vi "Main_PC.vi"() -> ()   [LabVIEW 2019]
uses:
  <vilib>/myRIO/Instrument Drivers/Onboard IO/UART/typedef/VISA Configuration.ctl
  <vilib>/Instr/_visa.llb/VISA Configure Serial Port (Instr).vi
  <vilib>/myRIO/Instrument Drivers/Onboard IO/UART/UART.lvlib
panel:
  in  "VISA resource name":refnum<visa-resource-name>
  out "Drilling Process":string
  out "RollDetection":bool
  out "Ready to Fly":bool
  in  "stop":bool
  out "error out":errorcluster
  in  "error in (no error)":errorcluster
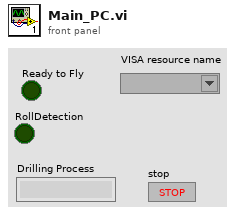
[diagram p1: front panel]
types:
  T1 = typedef "UART.lvlib/VISA Configuration.ctl" = cluster{"baud rate (9600)":u32, "data bits (8)":u16, "parity (0:none)":enum16{"None", "Odd", "Even", "Mark", "Space"}, "stop bits (10: 1 bit)":u16, "flow control (0:none)":u16, "termination char\n(0xA = '\\n' = LF) ":u8, "Enable Termination\nChar (T)":bool, "timeout (10sec)":u32}
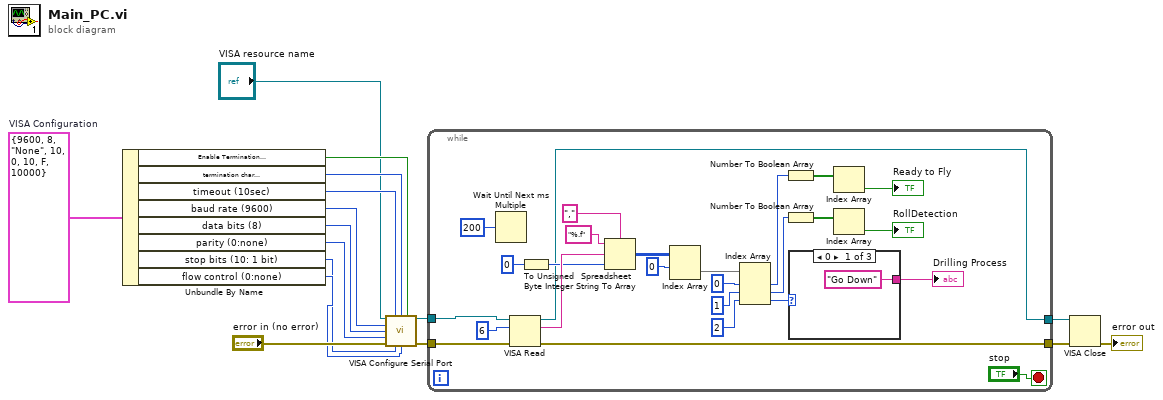
[diagram p0: block diagram]
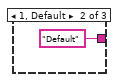
[diagram p2: hidden frame]
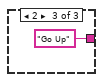
[diagram p3: hidden frame]
diagram:
  w4 = T1 {"baud rate (9600)"=9600, "data bits (8)"=8, "parity (0:none)"=enum."None", "stop bits (10: 1 bit)"=10, "flow control (0:none)"=0, "termination char\n(0xA = '\\n' = LF) "=10, "Enable Termination\nChar (T)"=FALSE, "timeout (10sec)"=10000}  # VISA Configuration
  n1 = Unbundle By Name(w4) -> ("Enable Termination\nChar (T)"=w13:bool, "termination char\n(0xA = '\\n' = LF)"=w12:u8, "timeout (10sec)"=w11:u32, "baud rate (9600)"=w6:u32, "data bits (8)"=w7:u16, "parity (0:none)"=w8:enum16{"None", "Odd", "Even", "Mark", "Space"}, "stop bits (10: 1 bit)"=w9:u16, "flow control (0:none)"=w10:u16)
  n2 = call-poly "VISA Configure Serial Port"("VISA resource name"="VISA resource name", "timeout (10sec)"=w11, "termination char\n(0xA = '\\n' = LF)"=w12, "Enable Termination\nChar (T)"=w13, "baud rate (9600)"=w6, "data bits (8)"=w7, "parity (0:none)"=w8, "error in (no error)"="error in (no error)", "stop bits (10: 1 bit)"=w9, "flow control (0:none)"=w10) -> ("VISA resource name out"=w15:refnum<visa-resource-name>, "error out"=w14:errorcluster)  [unwired: 4 in]
  n3 = while {
    tunnel: w15 -> [w19]
    tunnel: w14 -> [w41]
    tunnel: [w40] -> w2
    tunnel: [w17] -> w3
    stop <- "stop" stop-if-true
    n4 = Wait Until Next ms Multiple(millisecond multiple=u32 200) -> ()  [unwired: 1 out]
    n5 = VISA Read(VISA resource name=w19, byte count=u32 6 ("Character Count"), error in (no error)=w41) -> (VISA resource name out=w17:refnum<visa-resource-name>, read buffer=w38:string, error out=w40:errorcluster)  [unwired: 1 out]
    n6 = To Unsigned Byte Integer(number=0) -> (unsigned 8bit integer=w35:u8)
    n7 = Spreadsheet String To Array(delimiter (Tab)=",", format string="%.f", spreadsheet string=w38, array type (2D Dbl)=w35) -> (array=w32:u8[][])
    n8 = Index Array(array=w32, index (row)=0) -> (element=w30:u8[])  [unwired: 1 in]
    n9 = Index Array(array=w30, index #1=0 ("index (row)"), index #2=1 ("index"), index #3=2 ("index")) -> (element #1=w27:u8, element #2=w23:u8, element #3=w21:u8)
    n10 = Number To Boolean Array(number=w27) -> (Boolean array=w26:bool[])
    n11 = Number To Boolean Array(number=w23) -> (Boolean array=w24:bool[])
    n12 = case shown="0" w21 {
      tunnel: ["Go Down" "Default" "Go Up"] -> w20
      frame 0 {
      }
      frame 1, Default {
      }
      frame 2 {
      }
    }
    "Drilling Process" <- w20
    n13 = Index Array(array=w26) -> (element=→"Ready to Fly":bool)  [unwired: 1 in]
    n14 = Index Array(array=w24) -> (element=→"RollDetection":bool)  [unwired: 1 in]
  }
  n15 = VISA Close(VISA resource name=w3, error in (no error)=w2) -> (error out=→"error out":errorcluster)
